vi "S2C_ExeScriptInit.vi"(8 "Error In":errorcluster, 11 "Q-Ref":refnum<queue>) -> (0 "Error Out":errorcluster)   [LabVIEW 2015]
doc: "Preforms pre-executions actions prior to calling the Run case."
uses:
  Globals/S2C_Globals.vi
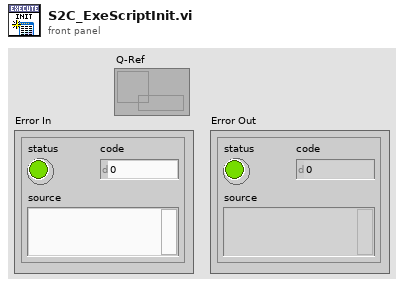
[diagram p1: front panel]
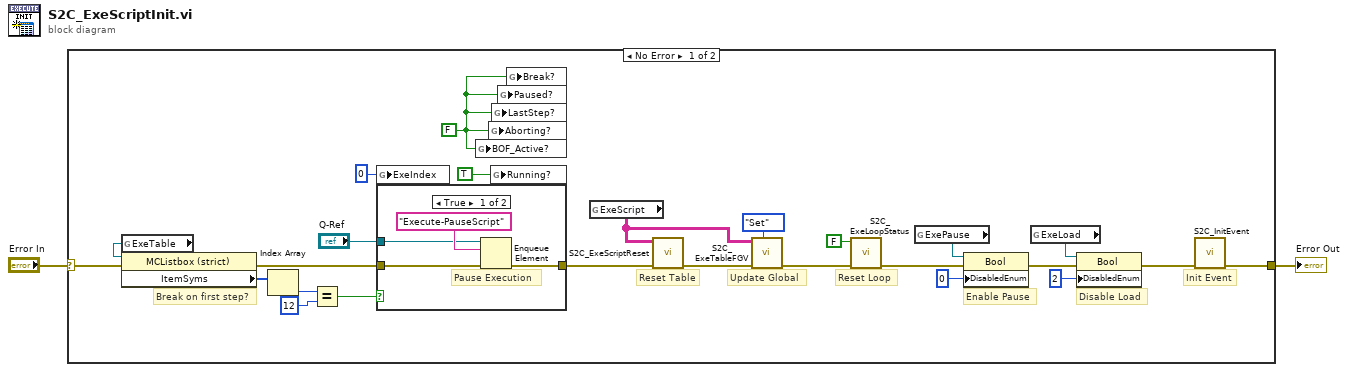
[diagram p0: block diagram]
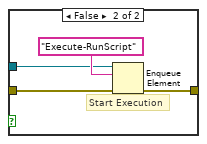
[diagram p2: hidden frame]
diagram:
  n1 = case shown="No Error" "Error In" {
    selector: "Error In" -> [w18 w36]
    tunnel: [w10 w36] -> w1
    frame No Error {
      w9 = FALSE ("Aborting?")
      # "Update Global"
      # "Init Event"
      # "Disable Load"
      # "Reset Loop"
      # "Break on first step?"
      # "Enable Pause"
      # "Reset Table"
      n2 = global read "S2C_Globals.vi" "ExeTable"() -> (w22:refnum<vi>)
      n3 = property class="MCListbox (strict)"(reference=w22, error in=w18) -> (error out=w16:errorcluster, "ItemSyms"=w19:i32[])  [unwired: 1 out]
      n4 = Index Array(array=w19) -> (element=w21:i32)  [unwired: 1 in]
      n5 = Equal?(x=w21, y=12) -> (x = y?=w17:bool)
      n6 = global write "S2C_Globals.vi" "ExeIndex"(0 ("ExeIndex")) -> ()
      n7 = case shown="True" w17 {
        tunnel: [w30 w34] -> w7
        tunnel: w16 -> [w29 w33]
        tunnel: "Q-Ref" -> [w28 w32]
        frame True {
          # "Pause Execution"
          n8 = Enqueue Element(queue=w28, element="Execute-PauseScript", error in (no error)=w29) -> (error out=w30:errorcluster)  [unwired: 1 in, 2 out]
        }
        frame False {
          # "Start Execution"
          n9 = Enqueue Element(queue=w32, element="Execute-RunScript", error in (no error)=w33) -> (error out=w34:errorcluster)  [unwired: 1 in, 2 out]
        }
      }
      n10 = global write "S2C_Globals.vi" "BOF_Active?"(w9) -> ()
      n11 = global write "S2C_Globals.vi" "Aborting?"(w9) -> ()
      n12 = global write "S2C_Globals.vi" "Running?"(TRUE ("Running?")) -> ()
      n13 = global write "S2C_Globals.vi" "LastStep?"(w9) -> ()
      n14 = global write "S2C_Globals.vi" "Paused?"(w9) -> ()
      n15 = global write "S2C_Globals.vi" "Break?"(w9) -> ()
      n16 = global read "S2C_Globals.vi" "ExeScript"() -> (w4:string[][])
      n17 = call "S2C_ExeScriptReset.vi"("Error In"=w7, "Script Data"=w4) -> ("Error Out"=w6:errorcluster)  [unwired: 9 in]
      n18 = call "S2C_ExeTableFGV.vi"("Action"=enum16{"Get", "Set"}."Set", "Error In"=w6, "Table In"=w4) -> ("Error Out"=w5:errorcluster)  [unwired: 7 in, 1 out]
      n19 = call "S2C_ExeLoopStatus.vi"("Error In"=w5, "Reset?"=FALSE) -> ("Error Out"=w14:errorcluster)  [unwired: 9 in]
      n20 = global read "S2C_Globals.vi" "ExePause"() -> (w24:refnum<vi>)
      n21 = property class="Bool"(reference=w24, error in=w14, "DisabledEnum"=u8 0) -> (error out=w11:errorcluster)  [unwired: 1 out]
      n22 = global read "S2C_Globals.vi" "ExeLoad"() -> (w12:refnum<vi>)
      n23 = property class="Bool"(reference=w12, error in=w11, "DisabledEnum"=u8 2) -> (error out=w3:errorcluster)  [unwired: 1 out]
      n24 = call "S2C_InitEvent.vi"("Error In"=w3) -> ("Error Out"=w10:errorcluster)  [unwired: 10 in]
    }
    frame Error {
    }
  }
  "Error Out" <- w1
